vi "Dictionary.vi"(0 "variant in":variant, 5 "key":string, 11 "error in":errorcluster, 13 "dict states":T1) -> (4 "variant out":variant, 15 "error out":errorcluster)   [LabVIEW 2021, in "Converter Reusables.lvlib"]
uses:
  Converter Reusables.lvlib
  TypeDefs/Dictionary States.ctl
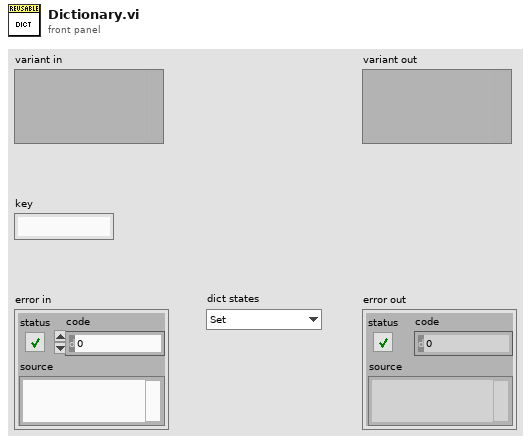
[diagram p1: front panel]
types:
  T1 = typedef "Converter Reusables.lvlib/Dictionary States.ctl" = enum16{"Set", "Get", "Delete", "Delete All"}
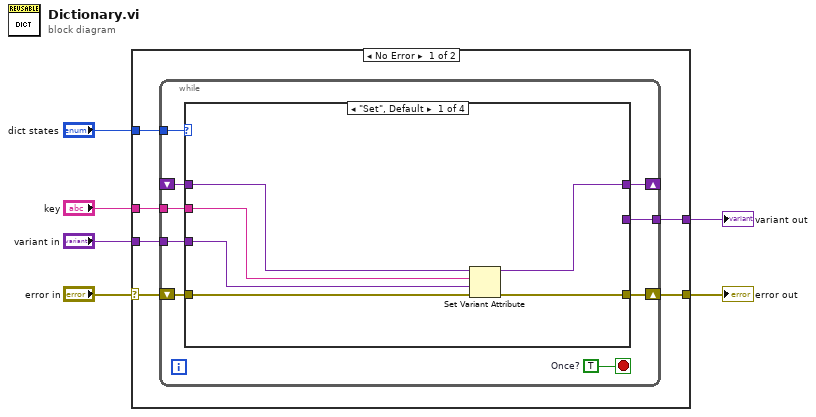
[diagram p0: block diagram]
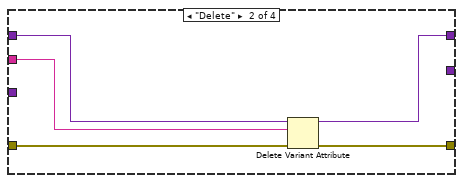
[diagram p2: hidden frame]
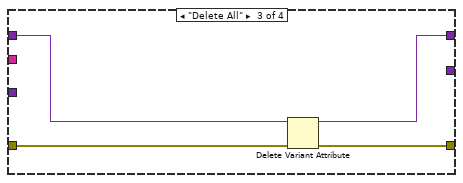
[diagram p3: hidden frame]
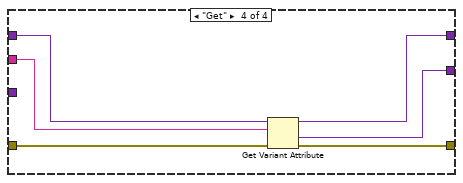
[diagram p4: hidden frame]
diagram:
  n1 = case shown="No Error" "error in" {
    selector: "error in" -> [w8 w43]
    tunnel: "variant in" -> [w12 _]
    tunnel: "key" -> [w11 _]
    tunnel: [w10 _] -> w6
    tunnel: "dict states" -> [w9 _]
    tunnel: [w7 w43] -> w5
    frame No Error {
      n2 = while {
        shift-right: [w20] -> _
        shift-left: _ -> [w21]
        tunnel: w12 -> [w19]
        tunnel: w11 -> [w18]
        tunnel: [w17] -> w10
        tunnel: w9 -> [w16]
        shift-right: [w13] -> w7
        shift-left: w8 -> [w15]
        stop <- w14 stop-if-true
        w14 = TRUE  # Once?
        n3 = case shown="\"Set\", Default" w16 {
          tunnel: w21 -> [w27 w32 w36 w42]
          tunnel: [w25 w31 w35 w41] -> w20
          tunnel: w19 -> [w26 _ _ _]
          tunnel: w18 -> [w24 w28 _ w37]
          tunnel: [_ _ _ w40] -> w17
          tunnel: w15 -> [w22 w29 w33 w39]
          tunnel: [w23 w30 w34 w38] -> w13
          frame "Set", Default {
            n4 = Set Variant Attribute(Variant=w27, name=w24, value=w26, error in=w22) -> (Variant out=w25:variant, error out=w23:errorcluster)  [unwired: 1 out]
          }
          frame "Delete" {
            n5 = Delete Variant Attribute(4:w29, 6:w28, 7:w32) -> (0:w30:errorcluster, 3:w31:variant)  [unwired: 1 out]
          }
          frame "Delete All" {
            n6 = Delete Variant Attribute(4:w33, 7:w36) -> (0:w34:errorcluster, 3:w35:variant)  [unwired: 1 in, 1 out]
          }
          frame "Get" {
            n7 = Get Variant Attribute(Variant=w42, name=w37, error in=w39) -> (duplicate Variant=w41:variant, value=w40:variant, error out=w38:errorcluster)  [unwired: 1 in, 1 out]
          }
        }
      }
    }
    frame Error {
    }
  }
  "error out" <- w5
  "variant out" <- w6
